vi "User Event Stop.vi"(8 "error in":errorcluster, 10 "event data":bool, 11 "Function":enum16{"Open", "Event Write", "Close"}(ring)) -> (0 "error out":errorcluster, 3 "Flag in":refnum<user-event>)   [LabVIEW 2016]
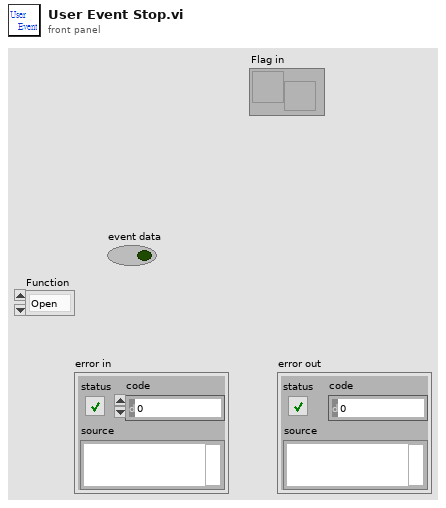
[diagram p1: front panel]
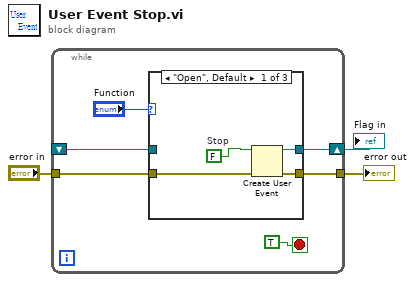
[diagram p0: block diagram]
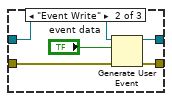
[diagram p2: hidden frame]
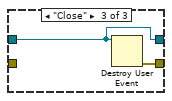
[diagram p3: hidden frame]
diagram:
  n1 = while {
    shift-right: [w7] -> w1
    shift-left: _ -> [w6]
    tunnel: "error in" -> [w5]
    tunnel: [w4] -> w2
    stop <- TRUE stop-if-true
    n2 = case shown="\"Open\", Default" "Function" {
      tunnel: [w13 w17 w19] -> w7
      tunnel: w6 -> [_ w18 w19]
      tunnel: w5 -> [w11 w16 _]
      tunnel: [w12 w15 w20] -> w4
      frame "Open", Default {
        w10 = FALSE  # Stop
        n3 = Create User Event(user event datatype=w10, error in=w11) -> (user event=w13:refnum<user-event>, error out=w12:errorcluster)
      }
      frame "Event Write" {
        n4 = Generate User Event(user event=w18, event data cluster="event data", error in=w16) -> (user event out=w17:refnum<user-event>, error out=w15:errorcluster)  [unwired: 1 in]
      }
      frame "Close" {
        n5 = Destroy User Event(user event=w19) -> (error out=w20:errorcluster)  [unwired: 1 in]
      }
    }
  }
  "error out" <- w2
  "Flag in" <- w1
